vi "Scenario jsObject Array.vi"(6 "Validate Fields/Templates? (t)":bool=TRUE, 7 "Connection Refnum":T1, 8 "error in (no error)":errorcluster, 9 "SCENARIOS (none)":T2[](array[typedef]), 10 "Scenarios jsObject Array Name (\"SCENARIOS\")":string="SCENARIOS", 11 "Previous String (\"\")":string) -> (0 "error out":errorcluster, 2 "Scenarios jsObject Array":string, 3 "SCENARIOS jsObject Definition":string, 5 "dup Connection Refnum":T1)   [LabVIEW 2011]
uses:
  Scenario Record.ctl
  Conditions/Condition Record.ctl
  Conditions/Condition Operators.ctl
  Summitek EXT/ODBC/SQL Controls/Connection Refnum.ctl
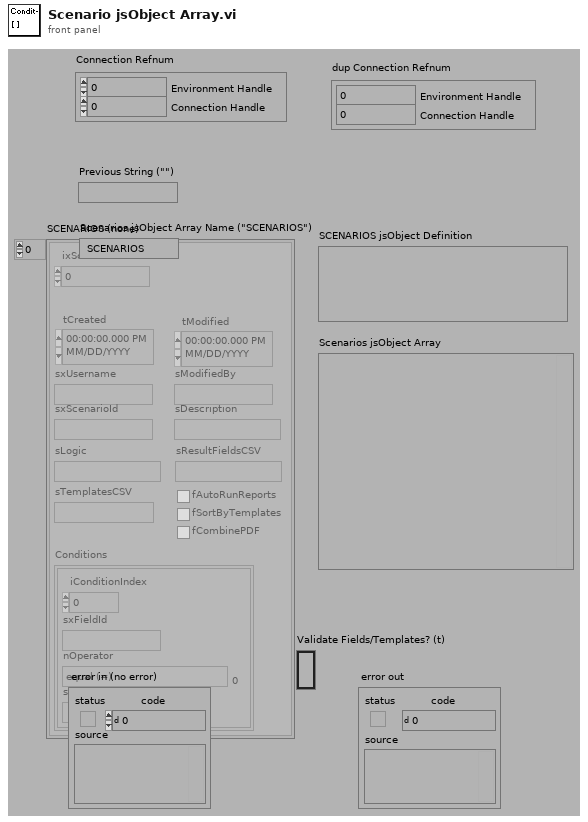
[diagram p1: front panel]
types:
  T1 = typedef "Connection Refnum.ctl" = cluster{"Environment Handle":i32, "Connection Handle":i32}
  T2 = typedef "Scenario Record.ctl" = cluster{"ixScenario":i32, "tCreated":timestamp, "tModified":timestamp, "sxUsername":string, "sModifiedBy":string, "sxScenarioId":string, "sDescription":string, "sLogic":string, "sResultFieldsCSV":string, "sTemplatesCSV":string, "fAutoRunReports":bool, "fSortByTemplates":bool, "fCombinePDF":bool, "Conditions":T3[]}
  T3 = typedef "Condition Record.ctl" = cluster{"iConditionIndex":i32, "sxFieldId":string, "nOperator":T4, "sMatchValue":string}
  T4 = typedef "Condition Operators.ctl" = enum16{"equal (=)", "not equal (\\u2260)", "less than (<)", "less than or equal (\\u2264)", "greater than (>)", "greater than or equal (\\u2265)", "contains", "does not contain"}
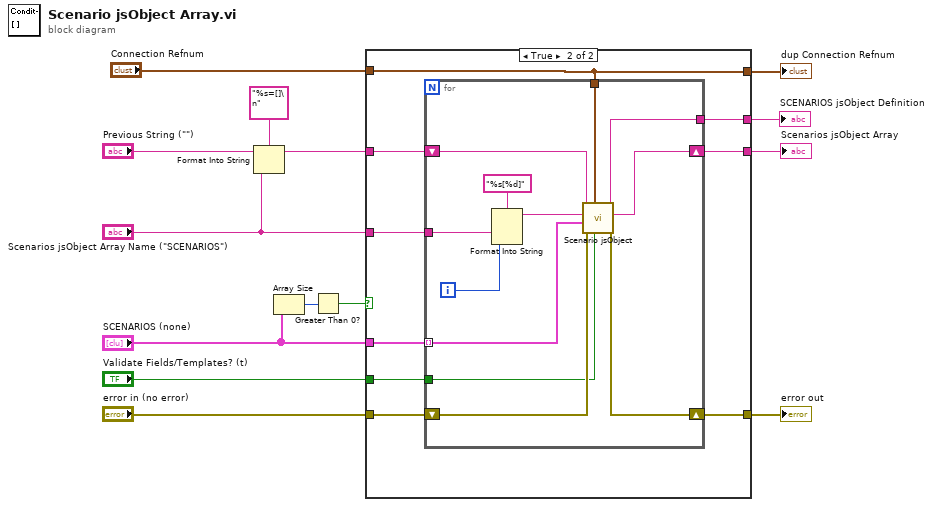
[diagram p0: block diagram]
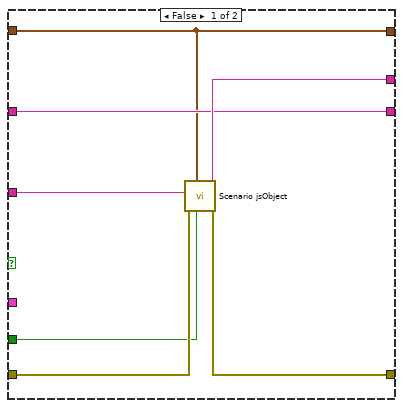
[diagram p2: hidden frame]
diagram:
  n1 = Format Into String(format string="%s=[]\n", initial string="Previous String (\"\")", "Scenarios jsObject Array Name (\"SCENARIOS\")") -> (resulting string=w13:string)  [unwired: 1 in, 1 out]
  n2 = Array Size(array="SCENARIOS (none)") -> (size(s)=w5:i32)
  n3 = Greater Than 0?(x=w5) -> (x > 0?=w4:bool)
  n4 = case shown="True" w4 {
    tunnel: w13 -> [w17 w30]
    tunnel: "error in (no error)" -> [w21 w29]
    tunnel: [w17 w28] -> w10
    tunnel: [w20 w27] -> w9
    tunnel: "Scenarios jsObject Array Name (\"SCENARIOS\")" -> [w18 w26]
    tunnel: [w19 w25] -> w7
    tunnel: "SCENARIOS (none)" -> [_ w24]
    tunnel: "Connection Refnum" -> [w16 w23]
    tunnel: [w16 w23] -> w2
    tunnel: "Validate Fields/Templates? (t)" -> [w15 w22]
    frame False {
      n5 = call "Scenario jsObject.vi"("Validate Fields/Templates? (t)"=w15, "Connection Refnum"=w16, "error in (no error)"=w21, "Scenario jsObject Name (\"\")"=w18) -> ("error out"=w20:errorcluster, "SCENARIO jsObject Definition"=w19:string)  [unwired: 2 in, 4 out]
    }
    frame True {
      n6 = for {
        tunnel: w24 -> [w35] mode=indexing
        shift-right: [w33] -> w28
        shift-left: w30 -> [w42]
        shift-right: [w40] -> w27
        shift-left: w29 -> [w41]
        tunnel: w26 -> [w37]
        tunnel: [w34] -> w25
        tunnel: w23 -> [w32]
        tunnel: w22 -> [w31]
        i -> [w36]
        n7 = Format Into String(format string="%s[%d]", w37, w36) -> (resulting string=w38:string)  [unwired: 2 in, 1 out]
        n8 = call "Scenario jsObject.vi"("Validate Fields/Templates? (t)"=w31, "Connection Refnum"=w32, "error in (no error)"=w41, "Scenario Record (empty)"=w35, "Scenario jsObject Name (\"\")"=w38, "Previous String (\"\")"=w42) -> ("error out"=w40:errorcluster, "Scenario jsObject"=w33:string, "SCENARIO jsObject Definition"=w34:string)  [unwired: 3 out]
      }
    }
  }
  "Scenarios jsObject Array" <- w10
  "error out" <- w9
  "SCENARIOS jsObject Definition" <- w7
  "dup Connection Refnum" <- w2
